vi "copyImagesToDataDir2.vi"(8 "error in (no error)":errorcluster, 10 "ImagePaths in":path[](array[path]), 11 "FileNeologist in":refnum<class "FileNeologist.lvclass">) -> (0 "error out":errorcluster, 2 "ImagePaths out":path[](array[path]), 3 "FileNeologist out":refnum<class "FileNeologist.lvclass">)   [LabVIEW 2009, in "Tools.lvlib" / "Filing.lvlib" / "FileNeologist.lvclass"]
uses:
  FileNeologist.lvclass
  FileNeologist.lvclass/FileNeologist.ctl
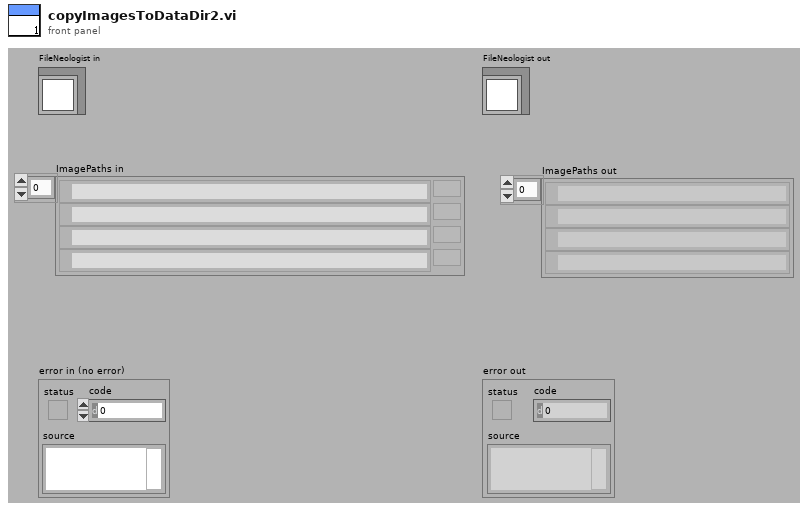
[diagram p1: front panel]
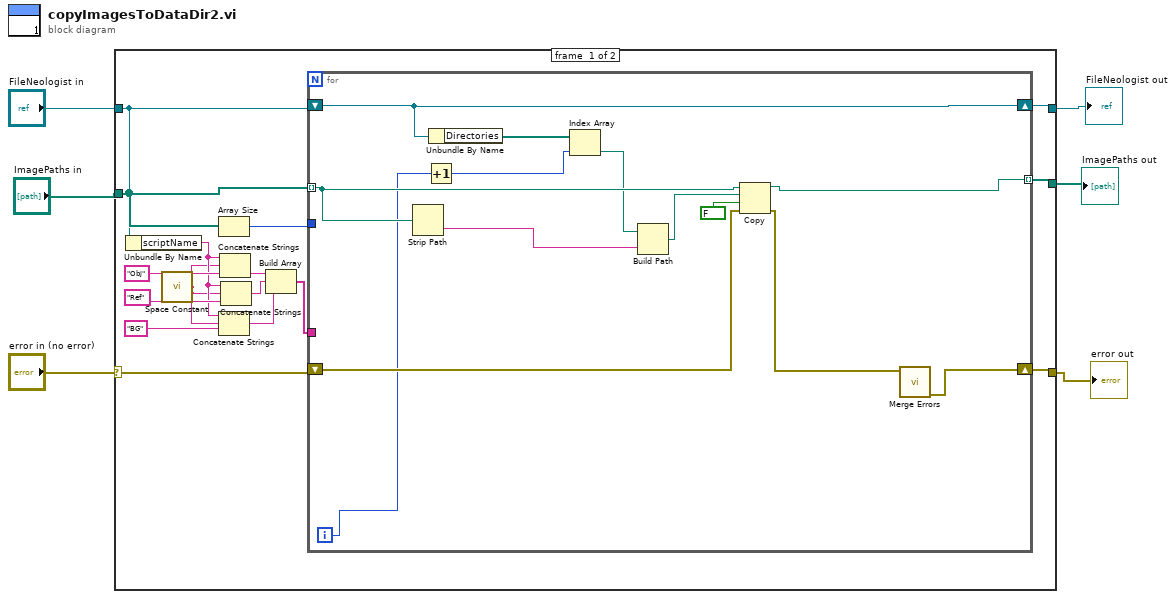
[diagram p0: block diagram]
diagram:
  n1 = case shown="No Error" "error in (no error)" {
    selector: "error in (no error)" -> [w19 w37]
    tunnel: [w21 w37] -> w3
    tunnel: [w20 w36] -> w4
    tunnel: "FileNeologist in" -> [w15 w36]
    tunnel: "ImagePaths in" -> [w17 _]
    tunnel: [w22 _] -> w1
    frame #0 {
      n2 = Unbundle By Name(w15) -> ("scriptName"=w9:string)
      n3 = call <vilib>:"Space Constant.vi"() -> ("String"=w7:string)
      n4 = Array Size(array=w17) -> (size(s)=w16:i32)
      n5 = Concatenate Strings(w9, w7, "BG") -> (w11:string)
      n6 = Concatenate Strings(w9, w7, "Obj") -> (w13:string)
      n7 = Concatenate Strings(w9, w7, "Ref") -> (w12:string)
      n8 = Build Array(w13, w12, w11) -> (w18:string[])
      n9 = for {
        tunnel: w17 -> [w35] mode=indexing
        tunnel: [w34] -> w22 mode=indexing
        shift-right: [w24] -> w20
        shift-left: w15 -> [w24]
        shift-right: [w33] -> w21
        shift-left: w19 -> [w32]
        tunnel: w18 -> [_]
        tunnel: w16 -> [_]
        i -> [w31]
        n10 = Strip Path(path=w35) -> (name=w23:string)  [unwired: 1 out]
        n11 = Increment(x=w31) -> (x+1=w25:i32)
        n12 = Unbundle By Name(w24) -> ("Directories"=w28:path[])
        n13 = Index Array(array=w28, index=w25) -> (element=w26:path)
        n14 = Build Path(base path=w26, name or relative path=w23) -> (appended path=w29:path)
        n15 = Copy(8:w32, 9:FALSE, 10:w29, 11:w35) -> (0:w27:errorcluster, 3:w34:path)  [unwired: 1 in, 1 out]
        n16 = call <vilib>:"Merge Errors.vi"("error in 1 (no error)"=w27) -> ("error out"=w33:errorcluster)  [unwired: 6 in]
      }
    }
    frame #1 {
    }
  }
  "error out" <- w3
  "FileNeologist out" <- w4
  "ImagePaths out" <- w1
